vi "Turn Button ON_OFF.vi"(8 "error in (no error)":errorcluster, 11 "Button in":refnum<class "Button.lvclass">) -> (0 "error out":errorcluster, 3 "Button out":refnum<class "Button.lvclass">)   [LabVIEW 2018, in "Button.lvclass"]
uses:
  Button.lvclass
  Button.lvclass/Button.ctl
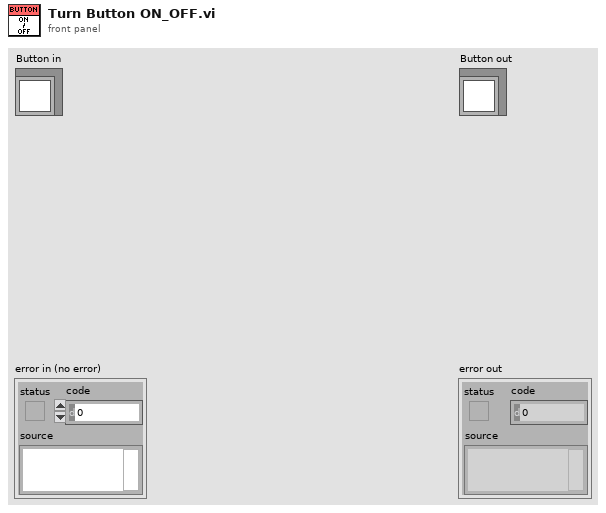
[diagram p1: front panel]
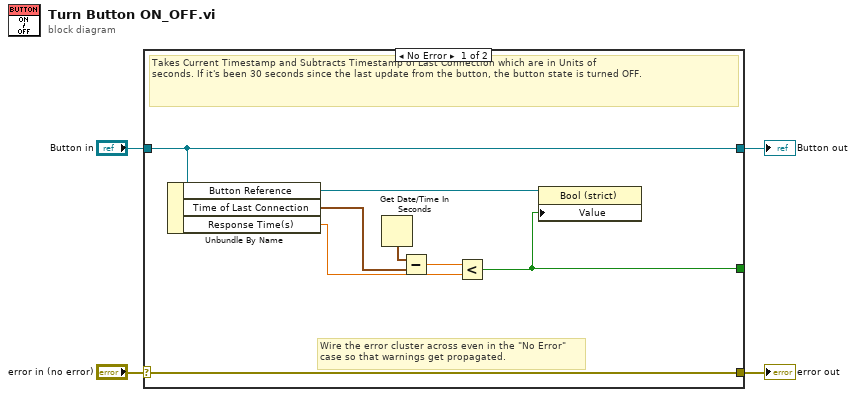
[diagram p0: block diagram]
diagram:
  n1 = case shown="No Error" "error in (no error)" {
    selector: "error in (no error)" -> [w12 w14]
    tunnel: [w12 w14] -> w3
    tunnel: [w11 w13] -> w1
    tunnel: "Button in" -> [w11 w13]
    tunnel: [w9 _] -> _
    frame No Error {
      # "Wire the error cluster across even in the \"No Error\"\ncase so that warnings get propagated."
      # "Takes Current Timestamp and Subtracts Timestamp of Last Connection which are in Units of \nseconds. If it's been 30 seconds since the last update from the button, the button state is turned OFF."
      n2 = Unbundle By Name(w11) -> ("Button Reference"=w10:refnum<vi>, "Time of Last Connection"=w6:timestamp, "Response Time(s)"=w5:dbl)
      n3 = Get Date/Time In Seconds() -> (seconds since 1Jan1904=w7:timestamp)
      n4 = Subtract(x=w7, y=w6) -> (x-y=w8:dbl)
      n5 = Less?(x=w8, y=w5) -> (x < y?=w9:bool)
      n6 = property class="Bool (strict)"(reference=w10, "Value"=w9) -> ()  [unwired: 1 in, 2 out]
    }
    frame Error {
    }
  }
  "error out" <- w3
  "Button out" <- w1
